vi "CRYFixed column width parse.vi"(10 "Data string":string, 11 "Fixed column width":i32) -> (3 "2D string array":string[][](array[string]))   [LabVIEW 2013]
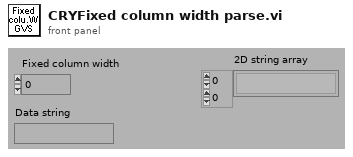
[diagram p1: front panel]
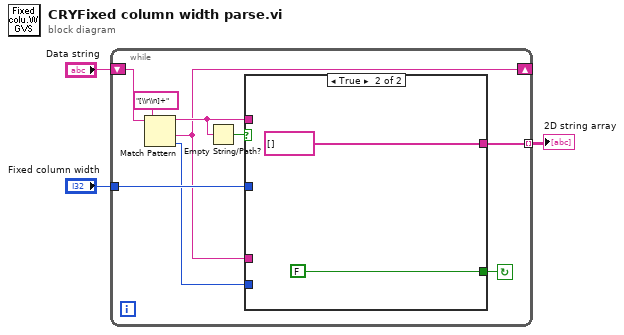
[diagram p0: block diagram]
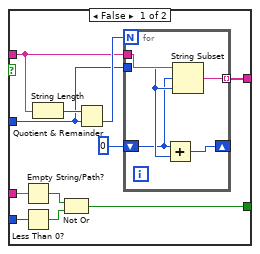
[diagram p2: hidden frame]
diagram:
  n1 = while {
    tunnel: [w9] -> w1 mode=indexing
    tunnel: "Fixed column width" -> [w10]
    shift-left: "Data string" -> [w11]
    shift-right: [w4] -> _
    stop <- w5 continue-if-true
    n2 = Match Pattern(string=w11, regular expression="[\\r\\n]+") -> (before substring=w8:string, after substring=w4:string, offset past match=w6:i32)  [unwired: 2 out]
    n3 = Empty String/Path?(string/path=w8) -> (empty?=w7:bool)
    n4 = case shown="True" w7 {
      tunnel: w10 -> [w21 _]
      tunnel: [w19 string[] []] -> w9
      tunnel: w8 -> [w18 _]
      tunnel: w6 -> [w17 _]
      tunnel: [w13 FALSE] -> w5
      tunnel: w4 -> [w16 _]
      frame False {
        n5 = Empty String/Path?(string/path=w16) -> (empty?=w15:bool)
        n6 = Less Than 0?(x=w17) -> (x < 0?=w14:bool)
        n7 = String Length(string=w18) -> (length=w23:i32)
        n8 = Not Or(1:w14, 2:w15) -> (0:w13:bool)
        n9 = Quotient & Remainder(x=w23, y=w21) -> (floor(x/y)=w22:i32)  [unwired: 1 out]
        n10 = for {
          N: w22 -> [_]
          shift-right: [w25] -> _
          shift-left: 0 -> [w26]
          tunnel: w18 -> [w28]
          tunnel: w21 -> [w27]
          tunnel: [w24] -> w19 mode=indexing
          n11 = Add(x=w26, y=w27) -> (x+y=w25:i32)
          n12 = String Subset(string=w28, offset (0)=w26, length (rest)=w27) -> (substring=w24:string)
        }
      }
      frame True {
      }
    }
  }
  "2D string array" <- w1
